vi "Read provider.vi"(8 "error in (no error)":errorcluster, 11 "Settings Service in":refnum<class "Settings Service.lvclass">) -> (0 "error out":errorcluster, 3 "provider":string)   [LabVIEW 2026, in "Settings Service.lvclass"]
uses:
  Settings Service.lvclass
  Settings Service.lvclass/Settings Service.ctl
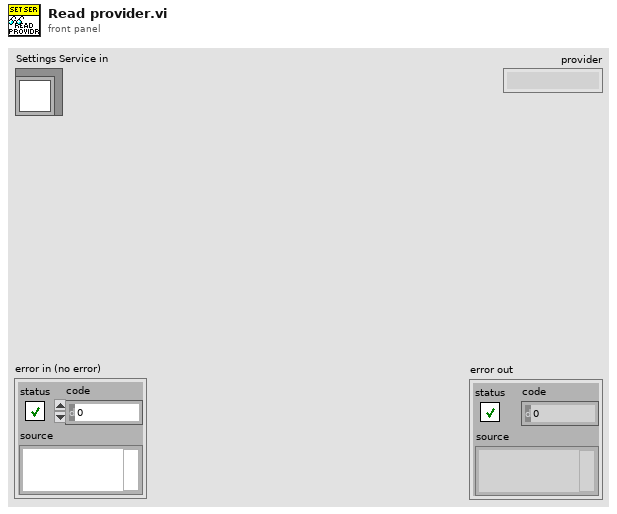
[diagram p1: front panel]
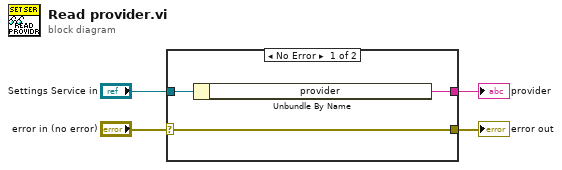
[diagram p0: block diagram]
diagram:
  n1 = case shown="No Error" "error in (no error)" {
    selector: "error in (no error)" -> [w7 w8]
    tunnel: [w7 w8] -> w3
    tunnel: "Settings Service in" -> [w6 _]
    tunnel: [w5 _] -> w1
    frame No Error {
      n2 = Unbundle By Name(w6) -> ("provider"=w5:string)
    }
    frame Error {
    }
  }
  "error out" <- w3
  "provider" <- w1
